vi "update string in array.vi"(9 "New Id":string, 10 "Old Id":string, 11 "registered modules":string[](array[string])) -> (3 "Array":string[](array[string]))   [LabVIEW 2013, in "engine configuration.lvclass"]
uses:
  engine configuration.lvclass
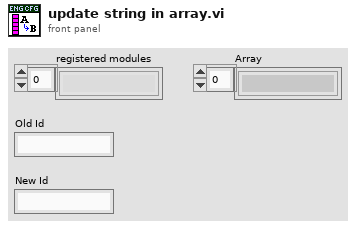
[diagram p1: front panel]
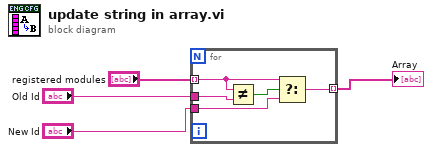
[diagram p0: block diagram]
diagram:
  n1 = for {
    tunnel: "registered modules" -> [w7] mode=indexing
    tunnel: [w6] -> w2 mode=indexing
    tunnel: "Old Id" -> [w8]
    tunnel: "New Id" -> [w5]
    n2 = Not Equal?(x=w7, y=w8) -> (x != y?=w9:bool)
    n3 = Select(t=w7, s=w9, f=w5) -> (s? t:f=w6:string)
  }
  "Array" <- w2
